vi "ChangeDate.vi"(8 "error in (no error)":errorcluster, 9 "Button":u16, 10 "Coords":T1, 11 "Calendar in":refnum<class "Calendar.lvclass">) -> (0 "error out":errorcluster, 3 "Calendar (dup)":refnum<class "Calendar.lvclass">)   [LabVIEW 2015, in "Calendar.lvclass"]
uses:
  Calendar.lvclass
  <vilib>/Utility/miscctls.llb/LVPoint32TypeDef.ctl
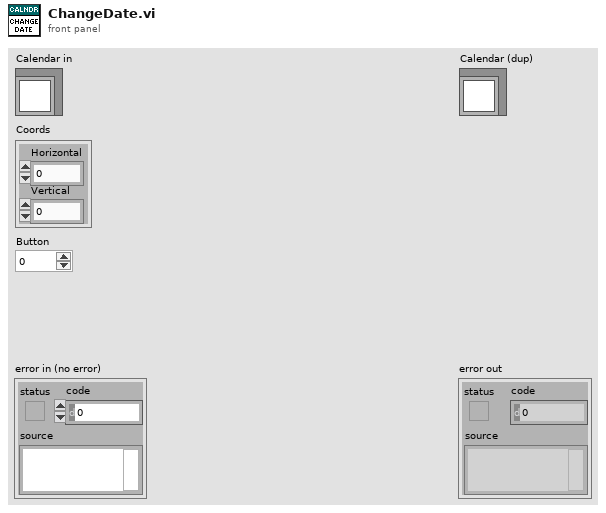
[diagram p1: front panel]
types:
  T1 = typedef "LVPoint32TypeDef.ctl" = cluster{"Horizontal":i32, "Vertical":i32}
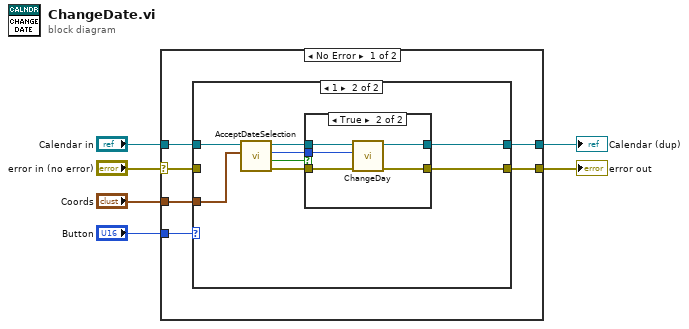
[diagram p0: block diagram]
diagram:
  n1 = case shown="No Error" "error in (no error)" {
    selector: "error in (no error)" -> [w7 w31]
    tunnel: [w8 w31] -> w5
    tunnel: [w9 w30] -> w3
    tunnel: "Calendar in" -> [w12 w30]
    tunnel: "Coords" -> [w11 _]
    tunnel: "Button" -> [w10 _]
    frame No Error {
      n2 = case shown="1" w10 {
        tunnel: w12 -> [w14 w22]
        tunnel: w11 -> [_ w21]
        tunnel: [w14 w16] -> w9
        tunnel: [w13 w15] -> w8
        tunnel: w7 -> [w13 _]
        frame Default {
        }
        frame 1 {
          n3 = call "AcceptDateSelection.vi"("Coords"=w21, "Calendar in"=w22) -> ("error out"=w18:errorcluster, "Accept?"=w19:bool, "Day of Month"=w17:i32, "Calendar (dup)"=w20:refnum<class "Calendar.lvclass">)  [unwired: 6 in]
          n4 = case shown="True" w19 {
            tunnel: w20 -> [w24 w29]
            tunnel: w18 -> [w23 w28]
            tunnel: w17 -> [_ w27]
            tunnel: [w24 w26] -> w16
            tunnel: [w23 w25] -> w15
            frame False {
            }
            frame True {
              n5 = call "ChangeDay.vi"("error in (no error)"=w28, "Day of Month"=w27, "Calendar in"=w29) -> ("error out"=w25:errorcluster, "Calendar (dup)"=w26:refnum<class "Calendar.lvclass">)  [unwired: 7 in]
            }
          }
        }
      }
    }
    frame Error {
    }
  }
  "error out" <- w5
  "Calendar (dup)" <- w3
